vi "Handle Command.vi"(8 "error in (no error)":errorcluster, 10 "CMD in":refnum<class "Update Speaker Vscale CMD.lvclass">, 11 "Object In":refnum<class>) -> (0 "error out":errorcluster, 1 "Command Successful?":bool, 2 "CMD out":refnum<class "Update Speaker Vscale CMD.lvclass">, 3 "Object Out":refnum<class>)   [LabVIEW 2017, in "gPAS Library.lvlib" / "Update Speaker Vscale CMD.lvclass"]
doc: "This VI will contain the code used to actually execute the request. If the request is successful, this will be indicated by the boolean output <b>Command Successful?</b>. The boolean output can then be used by the <b>Command Reply</b> which sends a reply if the reply queue is valid."
uses:
  Update Speaker Vscale CMD.lvclass
  nPAS.lvclass
  C:/Program Files (x86)/National Instruments/LabVIEW 2017/vi.lib/MSR Consulting, LLC/General Reuse/Instrument/Instrument.lvclass
  <vilib>/MSR Consulting, LLC/General Reuse/Instrument/Instrument.lvclass/Instrument.ctl
  nPAS.lvclass/nPAS.ctl
  Update Speaker Vscale CMD.lvclass/Update Speaker Vscale CMD.ctl
  <vilib>/MSR Consulting, LLC/General Reuse/Instrument/Read Log Session.vi
  Accessors/Read hFPGA.vi
  <vilib>/MSR Consulting, LLC/General Reuse/Instrument/Read ExtCom.vi
  <vilib>/Utility/error.llb/Error Cluster From Error Code.vi
  <vilib>/rvi/errors/niLvFpgaAdjustHostInterfaceError.vi
  <vilib>/MSR Consulting, LLC/General Reuse/Session APIs/_Session Fwk/Session - Root.lvclass
  <vilib>/rvi/interface/nirviReadWriteControl/nirviReadWriteControl.xnode
  FPGA Ref.ctl
  FPGA Bitfiles/server.lvbitx
  Session/Raw FPGA/FPGA Session.lvclass
  <vilib>/MSR Consulting, LLC/General Reuse/Session APIs/Session Log/System Log.lvclass
  NiFpgaLv.dll
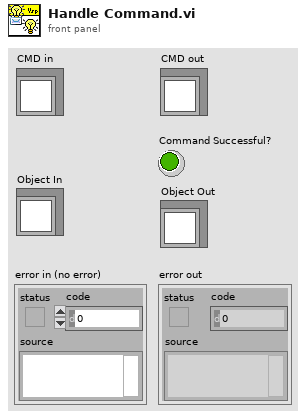
[diagram p1: front panel]
types:
  T1 = typedef "Session - Root.lvclass/Session Handle.ctl" = refnum<data-value>
  T2 = typedef "FPGA Ref.ctl" = refnum<k20>
  T3 = cluster{"tag":string, "section":string, "data":variant}
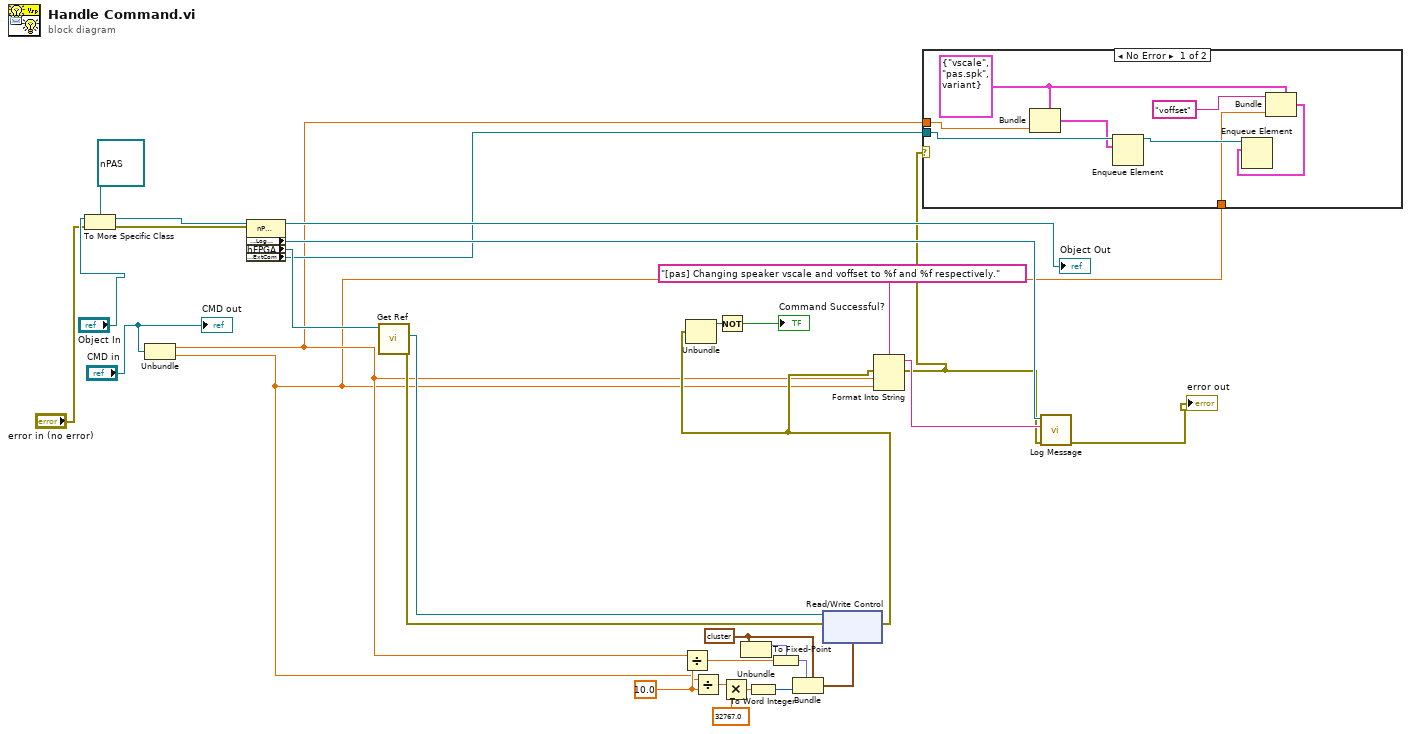
[diagram p0: block diagram]
diagram:
  w22 = sgl 10.0 ("y")
  w19 = cluster{"Vscale":fxp<+,32,0>, "Offset":i16} {"Vscale"=0.0, "Offset"=0} ("Speaker")
  n1 = To More Specific Class(target class=refnum<class "nPAS.lvclass"> refnum ("nPAS"), reference="Object In", error in="error in (no error)") -> (specific class reference=w30:refnum<class "nPAS.lvclass">, error out=w31:errorcluster)
  n2 = Unbundle("CMD in") -> (w2:dbl, w1:dbl)
  n3 = property class="nPAS"(reference=w30, error in=w31) -> (reference out=→"Object Out":refnum<class "nPAS.lvclass">, "Accessors:Log Session"=w10:T1, "hFPGA"=w26:T1, "Accessors:ExtCom"=w3:refnum<queue>)  [unwired: 1 out]
  n4 = call "Get Ref.vi"("Hanlde Out"=w26) -> ("error out"=w13:errorcluster, "FPGA Ref"=w15:T2)  [unwired: 8 in, 1 out]
  n5 = Divide(x=w2, y=w22) -> (x/y=w21:dbl)
  n6 = Divide(x=w1, y=w22) -> (x/y=w25:dbl)
  n7 = Multiply(x=w25, y=sgl 32767.0) -> (x*y=w23:dbl)
  n8 = Unbundle(w19) -> ("Vscale"=w20:fxp<+,32,0>)  [unwired: 1 out]
  n9 = To Word Integer(number=w23) -> (16bit integer=w17:i16)
  n10 = To Fixed-Point(fixed-point type=w20, number=w21) -> (fixed-point=w18:fxp<+,32,0>)
  n11 = Bundle(cluster=w19, "Vscale"=w18, "Offset"=w17) -> (w16:cluster{"Vscale":fxp<+,32,0>, "Offset":i16})
  n12 = xnode "Read/Write Control"("FPGA VI Reference In"=w15, "error in"=w13, "Speaker"=w16) -> ("error out"=w8:errorcluster)  [unwired: 1 out]
  n13 = Unbundle(w8) -> ("status"=w14:bool)  [unwired: 2 out]
  n14 = Not(x=w14) -> (.not. x?=→"Command Successful?":bool)
  n15 = Format Into String(format string="[pas] Changing speaker vscale and voffset to %f and %f respectively.", error in=w8, w2, w1) -> (resulting string=w7:string, error out=w4:errorcluster)  [unwired: 1 in]
  n16 = case shown="No Error" w4 {
    tunnel: w3 -> [w39 _]
    tunnel: w2 -> [w38 _]
    tunnel: w1 -> [w35 _]
    frame No Error {
      w33 = T3 {"tag"="vscale", "section"="pas.spk", "data"=variant} ("element")
      n17 = Bundle(cluster=w33, "data"=w38) -> (w37:T3)  [unwired: 2 in]
      n18 = Enqueue Element(queue=w39, element=w37) -> (queue out=w36:refnum<queue>)  [unwired: 2 in, 2 out]
      n19 = Bundle(cluster=w33, "tag"="voffset", "data"=w35) -> (w34:T3)  [unwired: 1 in]
      n20 = Enqueue Element(queue=w36, element=w34) -> ()  [unwired: 2 in, 3 out]
    }
    frame Error {
    }
  }
  n21 = call <vilib>:"Log Message.vi"("error in"=w4, "MSG In"=w7, "session in"=w10) -> ("error out"=→"error out":errorcluster)  [unwired: 7 in, 1 out]
  "CMD out" <- "CMD in"
